vi "Calculate_1Minute_Averages.vi"(0 "Current time":dbl) -> ()   [LabVIEW 2012]
uses:
  <vilib>/Analysis/baseanly.llb/Mean (DBL).vi
  <vilib>/Analysis/NI_AALBase.lvlib
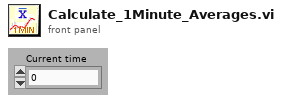
[diagram p1: front panel]
types:
  T1 = cluster{"Data out":dbl, "Data out":dbl, "Data out":dbl, "Data out":dbl, "Data out":dbl, "Data out":dbl, "Data out":dbl, "Data out":dbl, "Data out":dbl, "Data out":dbl, "Data out":dbl, "Data out":dbl, "Data out":dbl, "Data out":dbl, "seconds since 1Jan1904":dbl}
  T2 = cluster{"Data out":dbl, "Data out":dbl, "Data out":dbl, "Data out":dbl, "Data out":dbl, "Data out":dbl, "Data out":dbl, "Data out":dbl, "Data out":dbl, "Data out":dbl, "Data out":dbl, "Data out":dbl, "Data out":dbl, "Data out":dbl, "seconds since 1Jan1904":dbl}[]
  T3 = cluster{"mean":dbl, "mean":dbl, "mean":dbl, "mean":dbl, "mean":dbl, "mean":dbl, "mean":dbl, "mean":dbl, "mean":dbl, "mean":dbl, "mean":dbl, "mean":dbl, "mean":dbl, "mean":dbl, "mean":dbl}
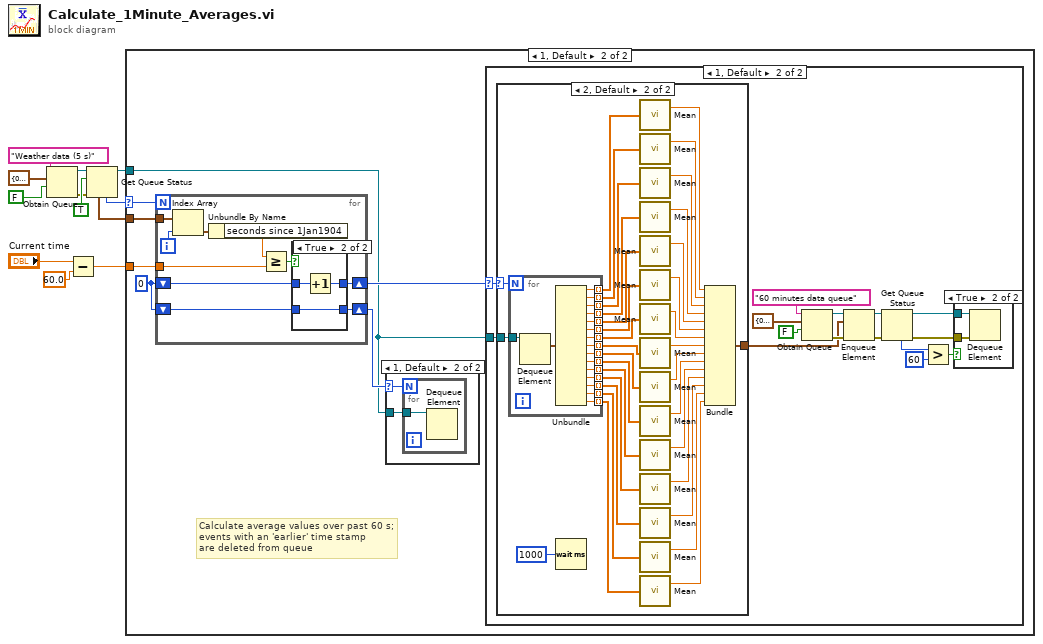
[diagram p0: block diagram]
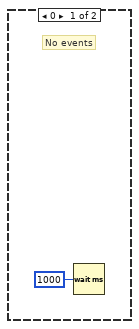
[diagram p2: hidden frame]
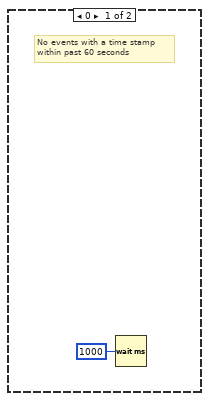
[diagram p4: hidden frame]
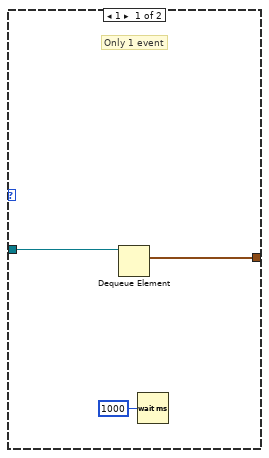
[diagram p6: hidden frame]
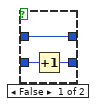
[diagram p7: hidden frame]
diagram:
  n1 = Obtain Queue(name (unnamed)="Weather data (5 s)", element data type=T1 {"Data out"=0.0, "Data out"=0.0, "Data out"=0.0, "Data out"=0.0, "Data out"=0.0, "Data out"=0.0, "Data out"=0.0, "Data out"=0.0, "Data out"=0.0, "Data out"=0.0, "Data out"=0.0, "Data out"=0.0, "Data out"=0.0, "Data out"=0.0, "seconds since 1Jan1904"=0.0} ("output cluster"), create if not found? (T)=FALSE) -> (queue out=w9:refnum<queue>, error out=w4:errorcluster)  [unwired: 2 in, 1 out]
  n2 = Subtract(x="Current time", y=60.0) -> (x-y=w2:dbl)
  n3 = Get Queue Status(queue=w9, return elements? (F)=TRUE, error in (no error)=w4) -> (queue out=w6:refnum<queue>, # elements in queue=w8:i32, elements=w7:T2)  [unwired: 5 out]
  n4 = case shown="1, Default" w8 {
    selector: w8 -> [_ w18]
    tunnel: w7 -> [_ w20]
    tunnel: w6 -> [_ w14]
    tunnel: w2 -> [_ w19]
    frame 0 {
      # "No events"
      n5 = Wait (ms)(milliseconds to wait=u32 1000) -> ()  [unwired: 1 out]
    }
    frame 1, Default {
      w16 = 0
      # "Calculate average values over past 60 s;\nevents with an 'earlier' time stamp\nare deleted from queue"
      n6 = for {
        N: w18 -> [_]
        tunnel: w20 -> [w105]
        shift-right: [w104] -> w17
        shift-left: w16 -> [w103]
        tunnel: w19 -> [w99]
        shift-right: [w97] -> w15
        shift-left: w16 -> [w96]
        i -> [w102]
        n7 = Index Array(array=w105, index=w102) -> (element=w101:T1)
        n8 = Unbundle By Name(w101) -> ("seconds since 1Jan1904"=w100:dbl)
        n9 = Greater Or Equal?(x=w100, y=w99) -> (x >= y?=w98:bool)
        n10 = case shown="True" w98 {
          tunnel: w103 -> [w108 w110]
          tunnel: [w108 w111] -> w104
          tunnel: [w107 w109] -> w97
          tunnel: w96 -> [w106 w109]
          frame False {
            n11 = Increment(x=w106) -> (x+1=w107:i32)
          }
          frame True {
            n12 = Increment(x=w110) -> (x+1=w111:i32)
          }
        }
      }
      n13 = case shown="1, Default" w15 {
        selector: w15 -> [_ w21]
        tunnel: w14 -> [_ w22]
        frame 0 {
          # "No events\nto remove"
        }
        frame 1, Default {
          n14 = for {
            N: w21 -> [_]
            tunnel: w22 -> [w23]
            n15 = Dequeue Element(queue=w23) -> ()  [unwired: 2 in, 4 out]
          }
        }
      }
      n16 = case shown="1, Default" w17 {
        selector: w17 -> [_ w39]
        tunnel: w14 -> [_ w27]
        frame 0 {
          # "No events with a time stamp\nwithin past 60 seconds"
          n17 = Wait (ms)(milliseconds to wait=u32 1000) -> ()  [unwired: 1 out]
        }
        frame 1, Default {
          n18 = case shown="2, Default" w39 {
            selector: w39 -> [_ w46]
            tunnel: w27 -> [w44 w48]
            tunnel: [w43 w47] -> w28
            frame 1 {
              # "Only 1 event"
              n19 = Dequeue Element(queue=w44) -> (element=w43:T1)  [unwired: 2 in, 3 out]
              n20 = Wait (ms)(milliseconds to wait=u32 1000) -> ()  [unwired: 1 out]
            }
            frame 2, Default {
              n21 = for {
                N: w46 -> [_]
                tunnel: [w95] -> w64 mode=indexing
                tunnel: [w94] -> w65 mode=indexing
                tunnel: [w93] -> w66 mode=indexing
                tunnel: [w92] -> w67 mode=indexing
                tunnel: [w91] -> w68 mode=indexing
                tunnel: [w90] -> w69 mode=indexing
                tunnel: [w89] -> w70 mode=indexing
                tunnel: [w88] -> w71 mode=indexing
                tunnel: [w87] -> w72 mode=indexing
                tunnel: [w86] -> w77 mode=indexing
                tunnel: [w85] -> w76 mode=indexing
                tunnel: [w82] -> w75 mode=indexing
                tunnel: [w84] -> w74 mode=indexing
                tunnel: [w83] -> w73 mode=indexing
                tunnel: [w81] -> w78 mode=indexing
                tunnel: w48 -> [w80]
                n22 = Dequeue Element(queue=w80) -> (element=w79:T1)  [unwired: 2 in, 3 out]
                n23 = Unbundle(w79) -> ("Data out"=w95:dbl, "Data out"=w94:dbl, "Data out"=w93:dbl, "Data out"=w92:dbl, "Data out"=w91:dbl, "Data out"=w90:dbl, "Data out"=w89:dbl, "Data out"=w88:dbl, "Data out"=w87:dbl, "Data out"=w86:dbl, "Data out"=w85:dbl, "Data out"=w82:dbl, "Data out"=w84:dbl, "Data out"=w83:dbl, "seconds since 1Jan1904"=w81:dbl)
              }
              n24 = Wait (ms)(milliseconds to wait=u32 1000) -> ()  [unwired: 1 out]
              n25 = call-poly <vilib>:"Mean.vi"("X"=w64) -> ("mean"=w50:dbl)  [unwired: 1 out]
              n26 = call-poly <vilib>:"Mean.vi"("X"=w65) -> ("mean"=w51:dbl)  [unwired: 1 out]
              n27 = call-poly <vilib>:"Mean.vi"("X"=w66) -> ("mean"=w52:dbl)  [unwired: 1 out]
              n28 = call-poly <vilib>:"Mean.vi"("X"=w67) -> ("mean"=w53:dbl)  [unwired: 1 out]
              n29 = call-poly <vilib>:"Mean.vi"("X"=w68) -> ("mean"=w54:dbl)  [unwired: 1 out]
              n30 = call-poly <vilib>:"Mean.vi"("X"=w69) -> ("mean"=w55:dbl)  [unwired: 1 out]
              n31 = call-poly <vilib>:"Mean.vi"("X"=w70) -> ("mean"=w56:dbl)  [unwired: 1 out]
              n32 = call-poly <vilib>:"Mean.vi"("X"=w71) -> ("mean"=w57:dbl)  [unwired: 1 out]
              n33 = call-poly <vilib>:"Mean.vi"("X"=w72) -> ("mean"=w58:dbl)  [unwired: 1 out]
              n34 = call-poly <vilib>:"Mean.vi"("X"=w77) -> ("mean"=w59:dbl)  [unwired: 1 out]
              n35 = call-poly <vilib>:"Mean.vi"("X"=w76) -> ("mean"=w60:dbl)  [unwired: 1 out]
              n36 = call-poly <vilib>:"Mean.vi"("X"=w75) -> ("mean"=w61:dbl)  [unwired: 1 out]
              n37 = call-poly <vilib>:"Mean.vi"("X"=w74) -> ("mean"=w62:dbl)  [unwired: 1 out]
              n38 = call-poly <vilib>:"Mean.vi"("X"=w73) -> ("mean"=w63:dbl)  [unwired: 1 out]
              n39 = call-poly <vilib>:"Mean.vi"("X"=w78) -> ("mean"=w49:dbl)  [unwired: 1 out]
              n40 = Bundle("mean"=w50, "mean"=w51, "mean"=w52, "mean"=w53, "mean"=w54, "mean"=w55, "mean"=w56, "mean"=w57, "mean"=w58, "mean"=w59, "mean"=w60, "mean"=w61, "mean"=w62, "mean"=w63, "mean"=w49) -> (w47:T3)  [unwired: 1 in]
            }
          }
          n41 = Obtain Queue(name (unnamed)="60 minutes data queue", element data type=T1 {"Data out"=0.0, "Data out"=0.0, "Data out"=0.0, "Data out"=0.0, "Data out"=0.0, "Data out"=0.0, "Data out"=0.0, "Data out"=0.0, "Data out"=0.0, "Data out"=0.0, "Data out"=0.0, "Data out"=0.0, "Data out"=0.0, "Data out"=0.0, "seconds since 1Jan1904"=0.0} ("output cluster"), create if not found? (T)=FALSE) -> (queue out=w31:refnum<queue>, error out=w32:errorcluster)  [unwired: 2 in, 1 out]
          n42 = Enqueue Element(queue=w31, element=w28, error in (no error)=w32) -> (queue out=w33:refnum<queue>, error out=w34:errorcluster)  [unwired: 1 in, 1 out]
          n43 = Get Queue Status(queue=w33, error in (no error)=w34) -> (queue out=w38:refnum<queue>, error out=w37:errorcluster, # elements in queue=w25:i32)  [unwired: 1 in, 5 out]
          n44 = Greater?(x=w25, y=60) -> (0:w36:bool)
          n45 = case shown="True" w36 {
            tunnel: w37 -> [_ w40]
            tunnel: w38 -> [_ w41]
            frame False {
            }
            frame True {
              n46 = Dequeue Element(queue=w41, error in (no error)=w40) -> ()  [unwired: 1 in, 4 out]
            }
          }
        }
      }
    }
  }
